vi "shift-register-plotter.vi"() -> ()   [LabVIEW 2020]
panel:
  in  "操作 (0:open)":T1(ring)
  in  "Output file path":path=path "practice_outputs"
  in  "停止":bool
  out "XYグラフ":cluster{dbl[], dbl[]}(graph)
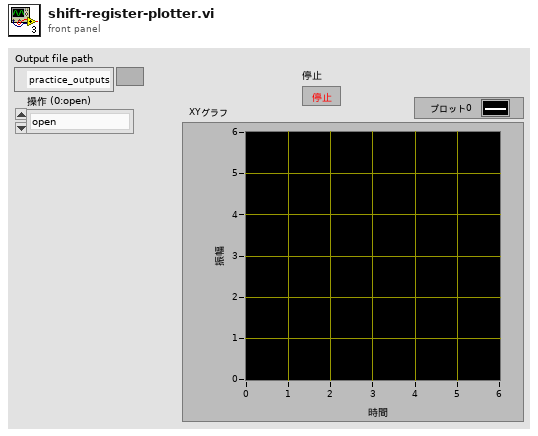
[diagram p1: front panel]
types:
  T1 = enum16{"open", "replace", "create", "open or create", "replace or create", "replace or create with confirmation"}
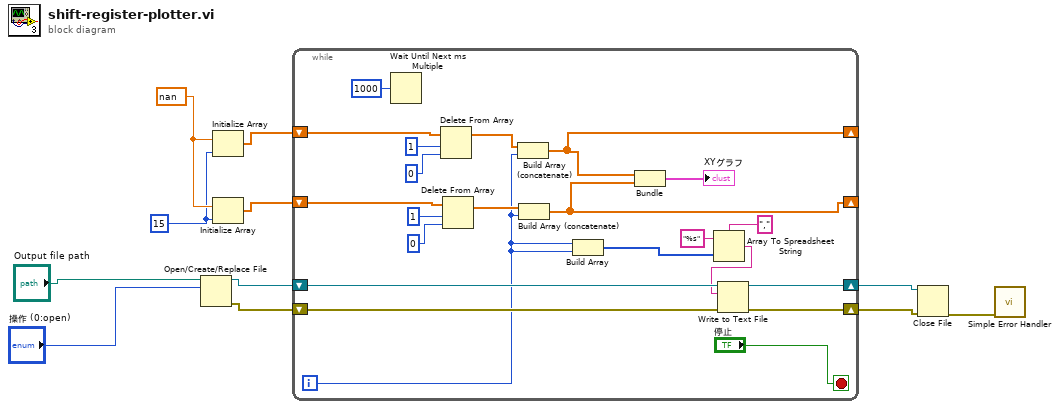
[diagram p0: block diagram]
diagram:
  w10 = 15
  w11 = nan
  n1 = Open/Create/Replace File(file path (use dialog)="Output file path", operation (0:open)="操作 (0:open)") -> (refnum out=w3:refnum<file>, error out=w5:errorcluster)  [unwired: 4 in, 1 out]
  n2 = Initialize Array(w11, w10) -> (w9:dbl[])
  n3 = Initialize Array(w11, w10) -> (w8:dbl[])
  n4 = while {
    shift-right: [w15] -> _
    shift-left: w9 -> [w31]
    shift-right: [w14] -> _
    shift-left: w8 -> [w28]
    shift-right: [w21] -> w4
    shift-left: w5 -> [w22]
    shift-right: [w19] -> w2
    shift-left: w3 -> [w20]
    i -> [w13]
    stop <- "停止" stop-if-true
    n5 = Wait Until Next ms Multiple(millisecond multiple=u32 1000 ("ミリ秒倍数")) -> ()  [unwired: 1 out]
    n6 = Delete From Array(array=w31, length=1 ("長さ"), index=0 ("指標")) -> (array with subset deleted=w27:dbl[])  [unwired: 1 out]
    n7 = Delete From Array(array=w28, length=1 ("長さ"), index=0 ("指標")) -> (array with subset deleted=w26:dbl[])  [unwired: 1 out]
    n8 = Build Array (concatenate)(w27, w13) -> (w15:dbl[])
    n9 = Build Array (concatenate)(w26, w13) -> (w14:dbl[])
    n10 = Build Array(w13, w13) -> (w12:i32[])
    n11 = Bundle(w15, w14) -> (→"XYグラフ":cluster{dbl[], dbl[]})  [unwired: 1 in]
    n12 = Array To Spreadsheet String(delimiter (Tab)="," ("デリミタ (タブ)"), array=w12, 3:"%s" ("形式文字列")) -> (spreadsheet string=w18:string)
    n13 = Write to Text File(file (use dialog)=w20, text=w18, error in=w22) -> (refnum out=w19:refnum<file>, error out=w21:errorcluster)  [unwired: 1 in, 1 out]
  }
  n14 = Close File(refnum=w2, error in=w4) -> (error out=w1:errorcluster)  [unwired: 1 out]
  n15 = call <vilib>:"Simple Error Handler.vi"("error in (no error)"=w1) -> ()  [unwired: 4 in, 5 out]
